vi "OxITC503 _Utility_ Check Command Response.vi"(2 "error in":errorcluster, 3 "read buffer":string) -> (0 "error out (no error)":errorcluster, 1 "Error occurred?":bool)   [LabVIEW 2014]
doc: "Checks the message returned by the device to the application after the reception of a remote command. It determines wheter an error response has been sent from the device: an error response consists of a \"?\" (question mark) followed by all or part of the command string in question.\n\nIf the device sends an ERROR RESPONSE \"Error occured?\" is set to True and \"error out\" will contain the error information."
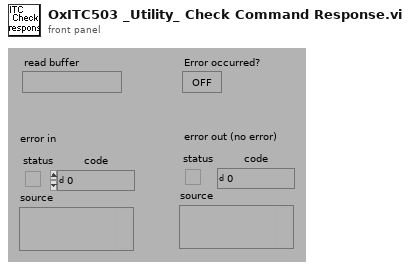
[diagram p1: front panel]
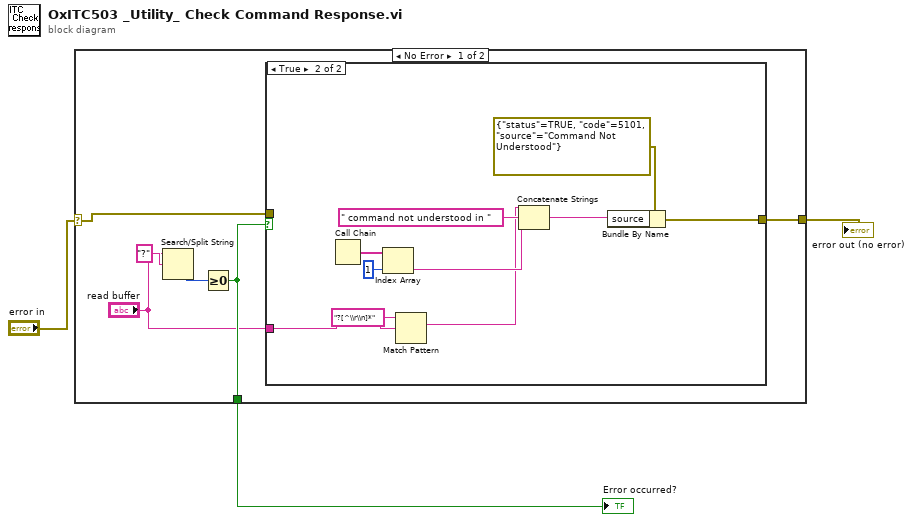
[diagram p0: block diagram]
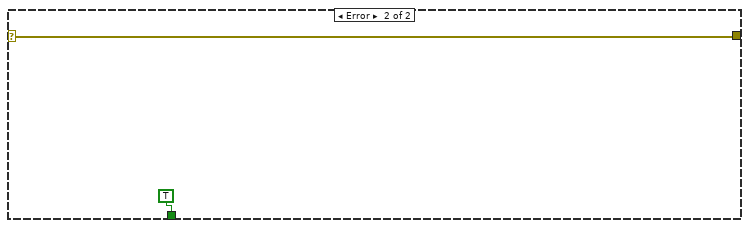
[diagram p3: hidden frame]
diagram:
  n1 = case shown="No Error" "error in" {
    selector: "error in" -> [w4 w22]
    tunnel: [w7 TRUE] -> w3
    tunnel: [w5 w22] -> w2
    frame No Error {
      n2 = Search/Split String(string="read buffer", search string/char (-)="?" ("search char (-)")) -> (offset of match=w8:i32)  [unwired: 1 in, 2 out]
      n3 = Greater Or Equal To 0?(x=w8) -> (x >= 0?=w7:bool)
      n4 = case shown="True" w7 {
        tunnel: "read buffer" -> [_ w13]
        tunnel: [w10 w11] -> w5
        tunnel: w4 -> [w10 _]
        frame False {
        }
        frame True {
          n5 = Call Chain() -> (call chain=w18:string[])
          n6 = Index Array(array=w18, index=1 ("Index")) -> (element=w16:string)
          n7 = Match Pattern(string=w13, regular expression="?[^\\r\\n]*") -> (match substring=w12:string)  [unwired: 1 in, 3 out]
          n8 = Concatenate Strings(w12, " command not understood in " ("Substring"), w16) -> (w15:string)
          n9 = Bundle By Name(cluster=errorcluster {"status"=TRUE, "code"=5101, "source"="Command Not Understood"} ("t"), "source"=w15) -> (w11:errorcluster)
        }
      }
    }
    frame Error {
    }
  }
  "Error occurred?" <- w3
  "error out (no error)" <- w2
